vi "Untitled 1.vi"() -> ()   [LabVIEW 2020]
panel:
  out "data":i8[](array[numeric])
  in  "file path (use dialog)":path
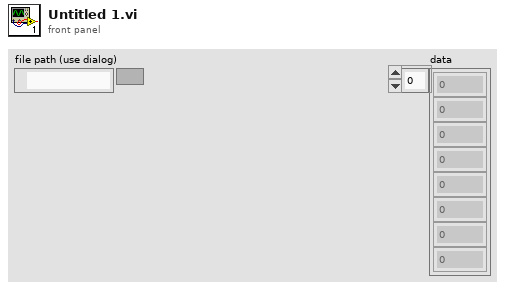
[diagram p1: front panel]
types:
  T1 = enum16{"big-endian, network order", "native, host order", "little-endian"}
  T2 = enum16{"open", "replace", "create", "open or create", "replace or create", "replace or create with confirmation"}
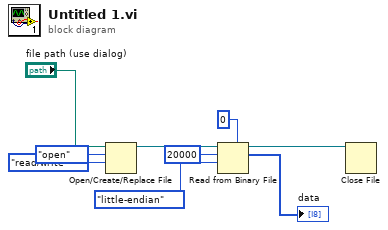
[diagram p0: block diagram]
diagram:
  n1 = Open/Create/Replace File(file path (use dialog)="file path (use dialog)", operation (0:open)=T2."open", access (0:read/write)=enum16{"read/write", "read-only", "write-only"}."read/write") -> (refnum out=w8:refnum<file>)  [unwired: 3 in, 2 out]
  n2 = Read from Binary File(5:i8 0, 9:T1."little-endian" ("byte order (0:big-endian, network order)"), 10:20000 ("count (1)"), 11:w8) -> (2:→"data":i8[], 3:w9:refnum<file>)  [unwired: 2 in, 2 out]
  n3 = Close File(refnum=w9) -> ()  [unwired: 1 in, 2 out]
